vi "AbortMeasurement.vi"(8 "error in (no error)":errorcluster, 11 "PalmSens in":refnum<class "PalmSens.lvclass">) -> (0 "error out":errorcluster, 3 "PalmSens out":refnum<class "PalmSens.lvclass">)   [LabVIEW 2025, in "PalmSens.lvclass"]
uses:
  PalmSens.lvclass
  PalmSens.lvclass/PalmSens.ctl
  E:/PSCode/PalmSens_SDK/labview/PalmSens/Libraries/PalmSens.Core.Simplified.LabVIEW.dll
  Libraries/PalmSens.Core.Simplified.LabVIEW.dll
panel:
  out "Is Measuring Refnum":refnum<vi>
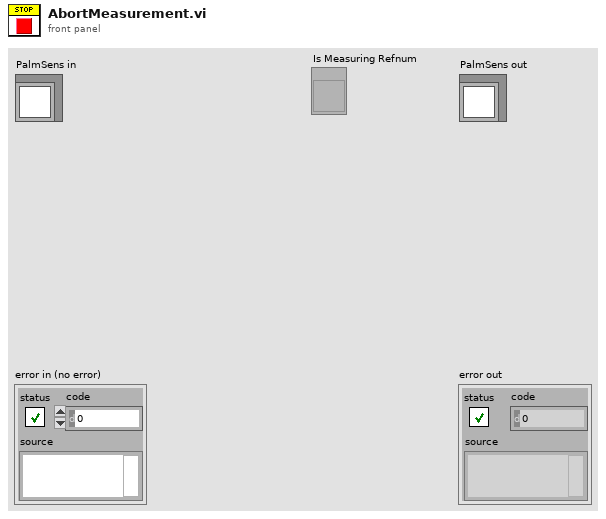
[diagram p1: front panel]
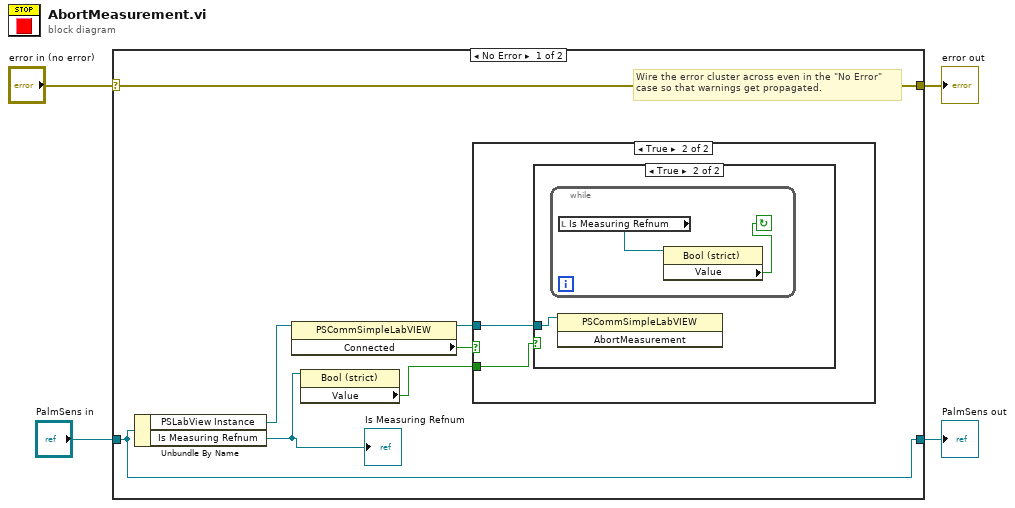
[diagram p0: block diagram]
diagram:
  n1 = case shown="No Error" "error in (no error)" {
    selector: "error in (no error)" -> [w11 w18]
    tunnel: [w11 w18] -> w3
    tunnel: [w7 w17] -> w1
    tunnel: "PalmSens in" -> [w7 w17]
    frame No Error {
      # "Wire the error cluster across even in the \"No Error\"\ncase so that warnings get propagated."
      n2 = Unbundle By Name(w7) -> ("PSLabView Instance"=w10:refnum<k24>, "Is Measuring Refnum"=w5:refnum<vi>)
      "Is Measuring Refnum" <- w5
      n3 = property class="PSCommSimpleLabVIEW"(reference=w10) -> (reference out=w8:refnum<k24>, "Connected"=w9:bool)  [unwired: 1 in, 1 out]
      n4 = property class="Bool (strict)"(reference=w5) -> ("Value"=w6:bool)  [unwired: 1 in, 2 out]
      n5 = case shown="True" w9 {
        tunnel: w8 -> [_ w13]
        tunnel: w6 -> [_ w12]
        frame False {
        }
        frame True {
          n6 = case shown="True" w12 {
            tunnel: w13 -> [_ w14]
            frame False {
            }
            frame True {
              n7 = while {
                stop <- w15 continue-if-true
                n8 = local read "Is Measuring Refnum"() -> (w16:refnum<vi>)
                n9 = property class="Bool (strict)"(reference=w16) -> ("Value"=w15:bool)  [unwired: 1 in, 2 out]
              }
              n10 = invoke class="PSCommSimpleLabVIEW" method="AbortMeasurement"(reference=w14) -> ()  [unwired: 2 in, 3 out]
            }
          }
        }
      }
    }
    frame Error {
    }
  }
  "error out" <- w3
  "PalmSens out" <- w1
